vi "TEST - Array of VData to VCluster.vi"(8 "error in (no error)":errorcluster) -> (0 "error out":errorcluster, 2 "pass":bool)   [LabVIEW 2020, in "test_openg_array.lvlib"]
uses:
  test_openg_array.lvlib
  <userlib>/_OpenG.lib/error/error.llb/openg_error.lvlib
  source/library/openg_variant.lvlib
panel:
  out "expected result":errorcluster
  out "result":errorcluster
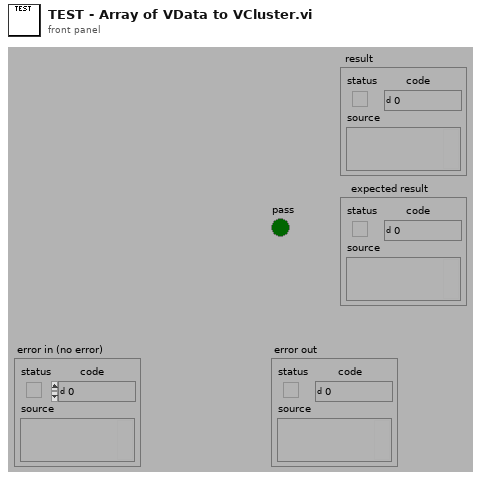
[diagram p1: front panel]
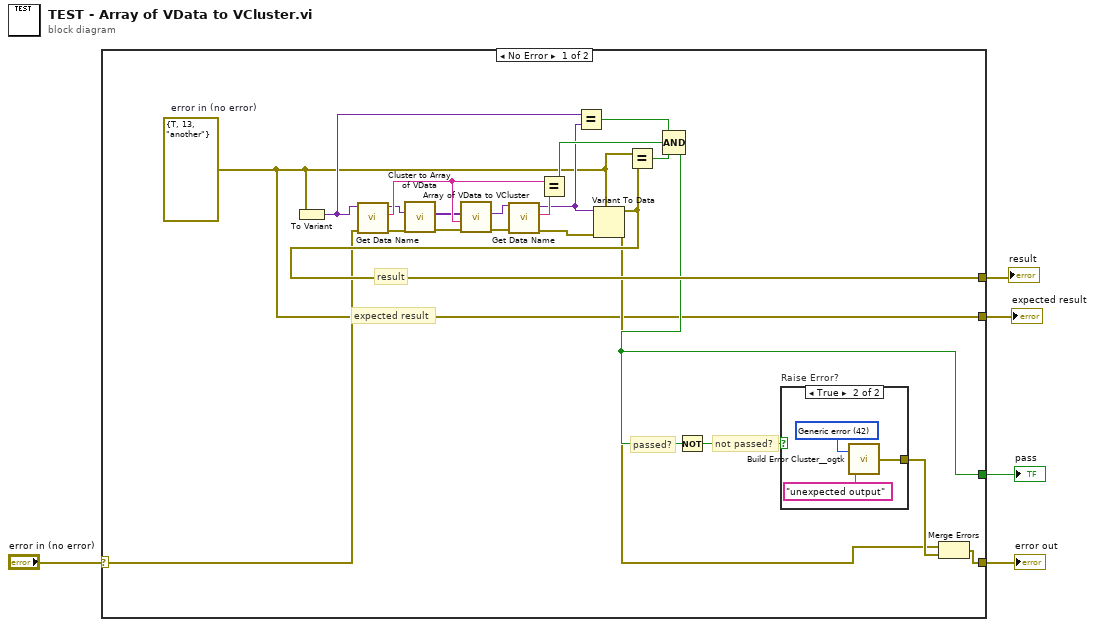
[diagram p0: block diagram]
diagram:
  n1 = case shown="No Error" "error in (no error)" {
    selector: "error in (no error)" -> [w18 w31]
    tunnel: [w21 _] -> w5
    tunnel: [w27 w31] -> w3
    tunnel: [w22 _] -> w2
    tunnel: [w6 _] -> w1
    frame No Error {
      w6 = errorcluster {"status"=TRUE, "code"=13, "source"="another"}  # error in (no error)
      # "result"
      # "expected result"
      # "not passed?"
      # "passed?"
      n2 = To Variant(anything=w6) -> (Variant=w19:variant)
      n3 = call "Get Data Name.vi"("error in (no error)"=w18, "Data"=w19) -> ("error out"=w11:errorcluster, "Data Name"=w13:string, "Data dup"=w12:variant)  [unwired: 7 in]
      n4 = call "Cluster to Array of VData.vi"("error in (no error)"=w11, "Cluster"=w12) -> ("error out"=w9:errorcluster, "Array of VData"=w10:variant[])  [unwired: 8 in]
      n5 = call "Array of VData to VCluster.vi"("error in (no error)"=w9, "Cluster Name"=w13, "Array"=w10) -> ("error out"=w7:errorcluster, "VCluster"=w8:variant)  [unwired: 7 in]
      n6 = call "Get Data Name.vi"("error in (no error)"=w7, "Data"=w8) -> ("error out"=w17:errorcluster, "Data Name"=w16:string, "Data dup"=w14:variant)  [unwired: 7 in]
      n7 = Equal?(x=w13, y=w16) -> (x = y?=w15:bool)
      n8 = Equal?(x=w19, y=w14) -> (x = y?=w23:bool)
      n9 = Variant To Data(error in=w17, type=w6, Variant=w14) -> (data=w22:errorcluster, error out=w20:errorcluster)
      n10 = Equal?(x=w6, y=w22) -> (x = y?=w24:bool)
      n11 = Compound Arithmetic op=AND(w23, w15, w24) -> (w21:bool)
      n12 = Not(x=w21) -> (.not. x?=w25:bool)
      n13 = case "Raise Error?" shown="True" w25 {
        tunnel: [_ w28] -> w26
        frame False {
        }
        frame True {
          w29 = 42 items=["No error", "Argument error", "Memory is full", "Out of zone", "End of file", "File already open", "Generic file I/O error", "File not found", "File permission error", "Disk is full", "Duplicate path", "Too many files open", "System feature not enabled", "Resource file not found", "Cannot add resource", "Resource not found", "Image not found", "Image memory error", "Pen does not exist", "Config type invalid", "Config token not found", "Config parse error", "Config memory error", "Bad external code format", "Bad external code offset", "External code not present", "Null window", "Destroy window error", "Null menu", "Print aborted", "Bad print record", "Print driver error", "Windows error during printing", "Memory error during printing", "Print dialog error", "Generic print error", "Invalid device refnum", "Device not found", "Device parameter error", "Device unit error", "Cannot open device", "Device call aborted", "Generic error", "Cancelled by user", "Object ID too low", "Object ID too high", "Object not in heap", "Unknown heap", "Unknown object (invalid DefProc)", "Unknown object (DefProc not in table)", "Message out of range", "Invalid (null) method", "Unknown message", "Manager call not supported", "Bad address", "Network operation in progress", "Network operation timed out", "Connection is busy", "Network attribute not supported", "Network error", "Address in use", "System out of memory", "Connection aborted", "Connection refused", "Not connected", "Already connected", "Connection closed", "Initialization error (interapplication manager)", "Bad occurrence", "Wait on unbound occurrence handler", "Occurrence queue overflow", "Datalog type conflict", "Unused", "Unrecognized type (interapplication manager)", "Memory corrupt", "Failed to make temporary DLL", "Old CIN version", "Drag socket not found", "Failed to load drop-object", "Failed to register OLE object", "Failed to release OLE object", "Format specifier type mismatch", "Unknown format specifier", "Too few format specifiers", "Too many format specifiers", "Scan failed", "Newer CIN version", "Error converting to variant", "Runtime menu error", "Password tampered", "Variant attribute not found", "Incompatible variant data type", "Event data is not available", "Event Store is not present", "Occurrence is not found", "Event Queue is not created", "Event info is not available", "Refnum passed is NULL", "Error retrieving Class GUID", "Error retrieving CoClass GUID", "Error retrieving TypeLib GUID.", "Bad built application magic bytes.", "Specific driver is different from the specific driver associated with the Logical Name.", "There is no session opened to the class driver.", "Max Error", "MAX - Error with config objects", "MAX - Error loading configuration", "MAX - Group not supported"]
          n14 = call <userlib>:"Build Error Cluster__ogtk.vi"("String to Prepend to source (\"\")"="unexpected output" ("String to Prepend to source (\"\")"), "code"=w29) -> ("error out"=w28:errorcluster)
        }
      }
      n15 = Merge Errors(w20, w26) -> (w27:errorcluster)
    }
    frame Error {
    }
  }
  "pass" <- w5
  "error out" <- w3
  "result" <- w2
  "expected result" <- w1
